vi "InitializeDotMatrix_wtConflict1.vi"(1 "Frame-to-frame displ":dbl[][](array[numeric])) -> (0 "Dot matrix":i16[][](array[numeric]))   [LabVIEW 2013]
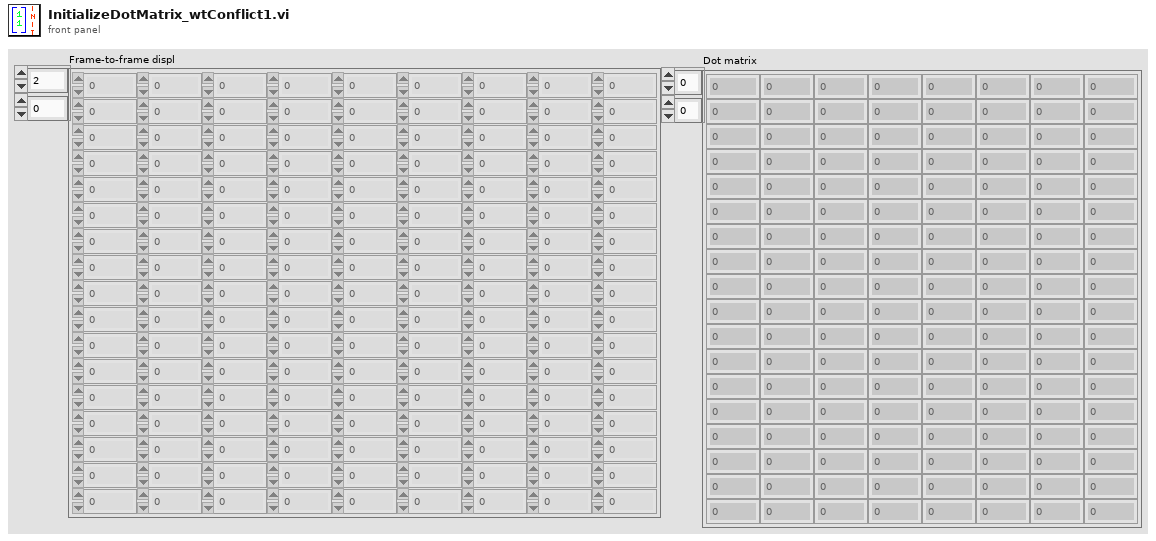
[diagram p1: front panel]
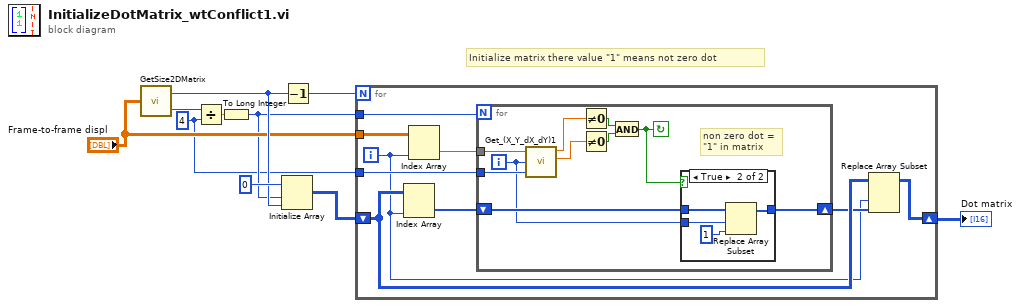
[diagram p0: block diagram]
diagram:
  w2 = 4 ("y")
  # "Initialize matrix there value \"1\" means not zero dot"
  n1 = call "GetSize2DMatrix.vi"("Array IN (2D)"="Frame-to-frame displ") -> ("# Cols"=w6:i32, "# Rows"=w8:i32)
  n2 = Divide(x=w8, y=w2) -> (x/y=w9:dbl)
  n3 = To Long Integer(number=w9) -> (32bit integer=w3:i32)
  n4 = Initialize Array(i16 0 ("element"), w3, w6) -> (w5:i16[][])
  n5 = Decrement(x=w6) -> (x-1=w10:i32)
  n6 = for {
    N: w10 -> [_]
    shift-right: [w12] -> w1
    shift-left: w5 -> [w14]
    tunnel: "Frame-to-frame displ" -> [w19]
    tunnel: w3 -> [w18]
    tunnel: w2 -> [w16]
    i -> [w11]
    n7 = Index Array(array=w14, index (col)=w11) -> (element=w15:i16[])  [unwired: 1 in]
    n8 = Index Array(array=w19, index (col)=w11) -> (element=w17:dbl[])  [unwired: 1 in]
    n9 = for {
      N: w18 -> [_]
      tunnel: w17 -> [w29]
      tunnel: w16 -> [w28]
      shift-right: [w20] -> w13
      shift-left: w15 -> [w22]
      i -> [w21]
      stop <- w23 continue-if-true
      # "non zero dot =\n\"1\" in matrix"
      n10 = call "Get_(X_Y_dX_dY)1.vi"("(X,Y,dX,dY)"=w29, "index"=w21, "multiplier"=w28) -> ("X"=w27:dbl, "Y"=w26:dbl)  [unwired: 2 out]
      n11 = Not Equal To 0?(x=w27) -> (x != 0?=w25:bool)
      n12 = Not Equal To 0?(x=w26) -> (x != 0?=w24:bool)
      n13 = And(x=w25, y=w24) -> (x .and. y?=w23:bool)
      n14 = case shown="True" w23 {
        tunnel: w22 -> [w30 w34]
        tunnel: w21 -> [_ w33]
        tunnel: [w30 w31] -> w20
        frame False {
        }
        frame True {
          n15 = Replace Array Subset(array=w34, new element=i16 1 ("new element/subarray"), index=w33) -> (w31:i16[])
        }
      }
    }
    n16 = Replace Array Subset(array=w14, new element=w13, index (col)=w11) -> (w12:i16[][])  [unwired: 1 in]
  }
  "Dot matrix" <- w1
